vi "Standby Power Slope.vi"(6 "Hours Index":i32=4, 8 "Error In":errorcluster, 9 "Power Index":i32=4, 10 "Loop Index":i32, 11 "15 Min Data Array":dbl[][](array[numeric])) -> (0 "Error Out":errorcluster, 3 "Slope (mW/hr)":dbl format="%.4f")   [LabVIEW 2018]
uses:
  <vilib>/Analysis/NI_AALPro.lvlib
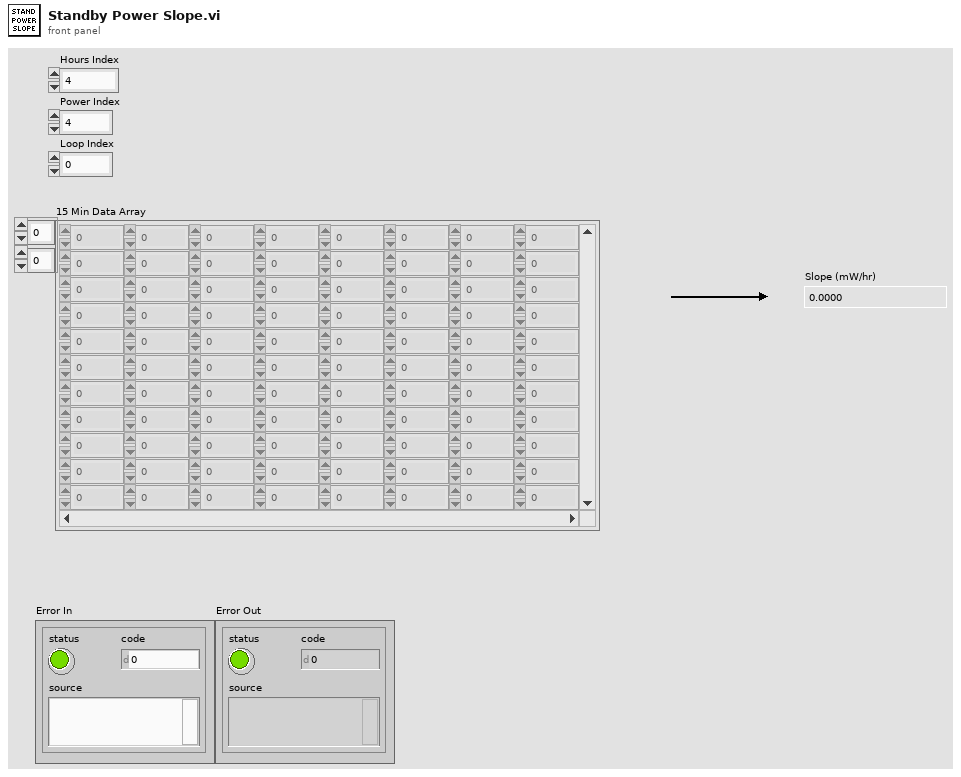
[diagram p1: front panel]
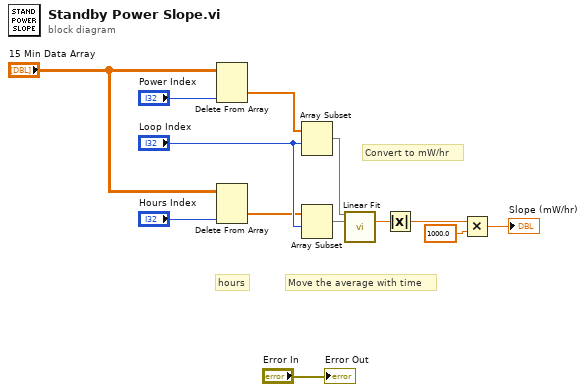
[diagram p0: block diagram]
diagram:
  # "Convert to mW/hr"
  # "hours"
  # "Move the average with time"
  n1 = Delete From Array(array="15 Min Data Array", index (col)="Power Index") -> (deleted portion=w9:dbl[])  [unwired: 2 in, 1 out]
  n2 = Delete From Array(array="15 Min Data Array", index (col)="Hours Index") -> (deleted portion=w10:dbl[])  [unwired: 2 in, 1 out]
  n3 = Array Subset(array=w9, index="Loop Index") -> (w2:dbl[])  [unwired: 1 in]
  n4 = Array Subset(array=w10, index="Loop Index") -> (w1:dbl[])  [unwired: 1 in]
  n5 = call <vilib>:"Linear Fit.vi"("Y"=w2, "X"=w1) -> ("slope"=w12:dbl)  [unwired: 9 in, 4 out]
  n6 = Absolute Value(x=w12) -> (abs(x)=w4:dbl)
  n7 = Multiply(x=w4, y=1000.0) -> (x*y=→"Slope (mW/hr)":dbl)
  "Error Out" <- "Error In"
